vi "NXT_MIDBRAIN Make Dummy Behavior Data.vi"(2 "Behavior #":i32, 3 "Behavior Weights":T1) -> (0 "Behavior Output":T2)   [LabVIEW 2012]
uses:
  behaviorOutput_t.ctl
  behaviorWeights_t.ctl
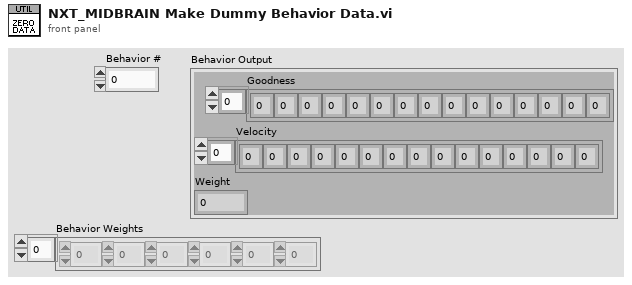
[diagram p1: front panel]
types:
  T1 = typedef "behaviorWeights_t.ctl" = i8[]
  T2 = typedef "behaviorOutput_t.ctl" = cluster{"Goodness":i8[], "Velocity":i8[], "Weight":i8}
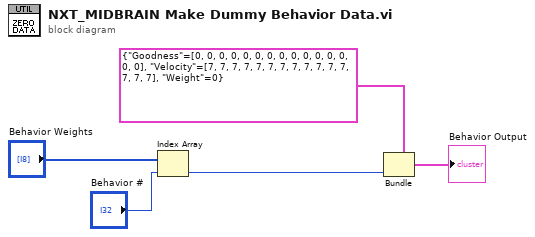
[diagram p0: block diagram]
diagram:
  n1 = Index Array(array="Behavior Weights", index="Behavior #") -> (element=w1:i8)
  n2 = Bundle(cluster=T2 {"Goodness"=[0, 0, 0, 0, 0, 0, 0, 0, 0, 0, 0, 0, 0, 0, 0], "Velocity"=[7, 7, 7, 7, 7, 7, 7, 7, 7, 7, 7, 7, 7, 7, 7], "Weight"=0} ("Behavior Output"), "Weight"=w1) -> (→"Behavior Output":T2)  [unwired: 2 in]
